vi "Cache.Get Transfers Group.vi"(10 "Transfer Group id":i32, 11 "Cache in":refnum<class "Cache.lvclass">) -> (2 "Transfers Group":refnum<class "Transfer Group.lvclass">, 3 "Cache out":refnum<class "Cache.lvclass">)   [LabVIEW 2017, in "DSF.Engine.lvlib" / "Cache.lvclass"]
uses:
  Cache.lvclass
  Transfer/Transfer Group.lvclass
  Cache.lvclass/Cache.ctl
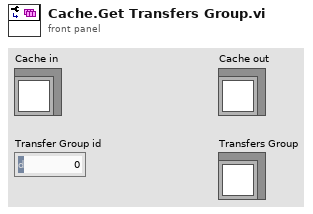
[diagram p1: front panel]
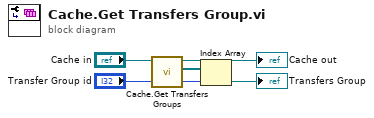
[diagram p0: block diagram]
diagram:
  n1 = call "Cache.Get Transfers Groups.vi"("Cache in"="Cache in") -> ("Transfers Groups"=w3:refnum<class "Transfer Group.lvclass">[], "Cache out"=→"Cache out":refnum<class "Cache.lvclass">)  [unwired: 9 in]
  n2 = Index Array(array=w3, index="Transfer Group id") -> (element=→"Transfers Group":refnum<class "Transfer Group.lvclass">)
